vi "UpdateRoiCache.vi"(8 "error in (no error)":errorcluster, 9 "Global Report":T1, 10 "roi cache in":variant, 11 "roi id":string) -> (0 "error out":errorcluster, 2 "roi cache out":variant)   [LabVIEW 2017, in "IrAnalysis.lvlib"]
uses:
  <vilib>/addons/InsightCM/Devices/Shared/Ir/IrAnalysis/IrAnalysis.lvlib
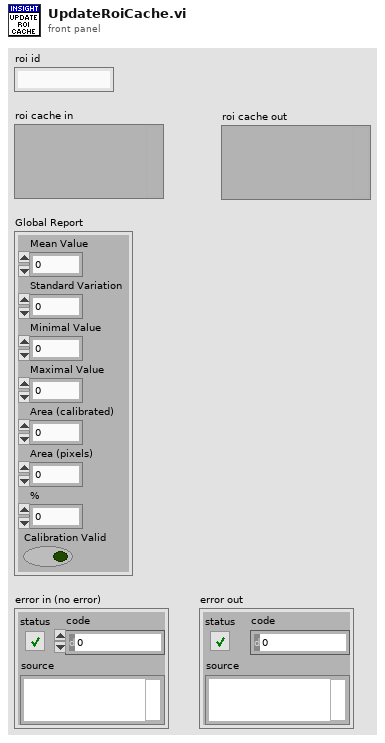
[diagram p1: front panel]
types:
  T1 = cluster{"Mean Value":sgl, "Standard Variation":sgl, "Minimal Value":sgl, "Maximal Value":sgl, "Area (calibrated)":sgl, "Area (pixels)":u32, "%":sgl, "Calibration Valid":bool}
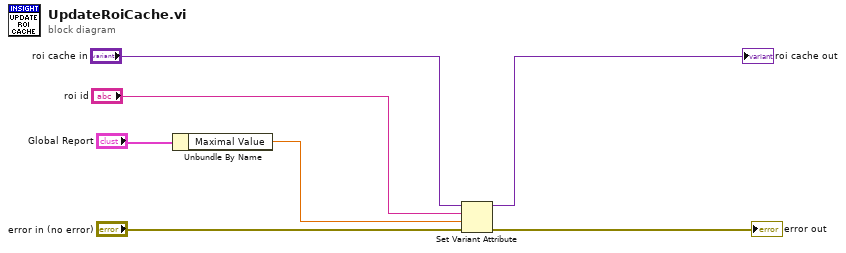
[diagram p0: block diagram]
diagram:
  n1 = Unbundle By Name("Global Report") -> ("Maximal Value"=w1:sgl)
  n2 = Set Variant Attribute(Variant="roi cache in", name="roi id", value=w1, error in="error in (no error)") -> (Variant out=→"roi cache out":variant, error out=→"error out":errorcluster)  [unwired: 1 out]
